vi "UTILITY Check Open TC.vi"(8 "Error In":errorcluster, 11 "Input TC Values":dbl[](array[numeric])) -> (0 "Error Out":errorcluster, 3 "Updated TC Array":string[](array[string]))   [LabVIEW 2018]
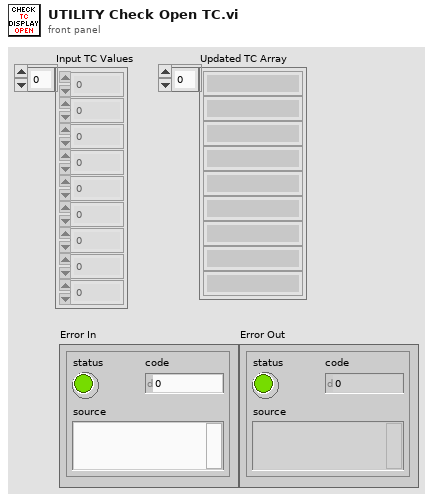
[diagram p1: front panel]
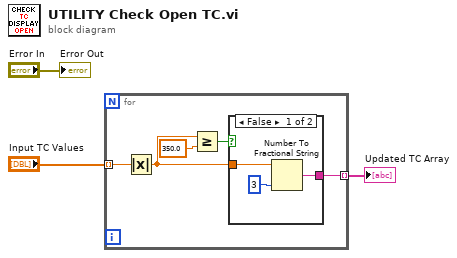
[diagram p0: block diagram]
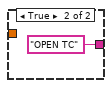
[diagram p2: hidden frame]
diagram:
  n1 = for {
    tunnel: "Input TC Values" -> [w5] mode=indexing
    tunnel: [w6] -> w2 mode=indexing
    n2 = Absolute Value(x=w5) -> (abs(x)=w4:dbl)
    n3 = Greater Or Equal?(x=w4, y=350.0) -> (x >= y?=w7:bool)
    n4 = case shown="False" w7 {
      tunnel: w4 -> [w10 _]
      tunnel: [w9 "OPEN TC"] -> w6
      frame False {
        n5 = Number To Fractional String(number=w10, precision (6)=i16 3) -> (F-format string=w9:string)  [unwired: 2 in]
      }
      frame True {
      }
    }
  }
  "Updated TC Array" <- w2
  "Error Out" <- "Error In"
